vi "Packet to String.vi"(11 "Data Packet":u8[](array[numeric])=[69, 48, 56, 95, 48, 48]) -> (3 "String":string)   [LabVIEW 2015, in "PAS.lvclass"]
uses:
  PAS.lvclass
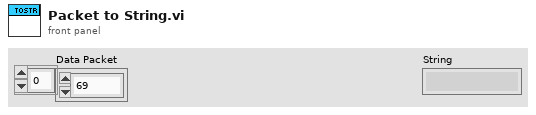
[diagram p1: front panel]
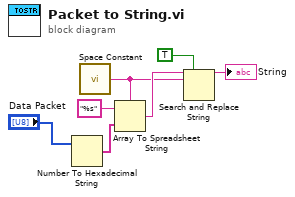
[diagram p0: block diagram]
diagram:
  n1 = Number To Hexadecimal String(2:"Data Packet") -> (0:w6:string[])  [unwired: 1 in]
  n2 = call <vilib>:"Space Constant.vi"() -> ("String"=w3:string)
  n3 = Array To Spreadsheet String(delimiter (Tab)=w3, array=w6, 3:"%s" ("format string")) -> (spreadsheet string=w4:string)
  n4 = Search and Replace String(replace all?=TRUE ("replace all? (F)"), input string=w4, search string=w3) -> (result string=→"String":string)  [unwired: 5 in, 3 out]
